vi "testAESDecryption-ECB-256.vi"(8 "error in (no error)":errorcluster, 11 "TestCase in":refnum<class "TestAES.lvclass">) -> (0 "error out":errorcluster, 3 "TestCase out":refnum<class "TestAES.lvclass">)   [LabVIEW 2021, in "TestAES.lvclass"]
uses:
  TestAES.lvclass
  C:/Program Files (x86)/National Instruments/LabVIEW 2021/vi.lib/addons/_JKI Toolkits/VI Tester/TestCase.llb/TestCase.lvclass
  TestAES.lvclass/TestAES.ctl
  <vilib>/addons/_JKI Toolkits/VI Tester/TestCase.llb/TestCase.lvclass
  <vilib>/Wiresmith Technology/VITAC (VI Tester Advanced Comparisons)/VITAC.lvlib
  Symmetric Encryption/dotNET Crypto Symmetric Encryption.lvlib
panel:
  out "Ciphertext in (hex)":string="Hello, World!"
  out "Key (hex)":string="01234567890"
  out "Expected plaintext (hex)":string
  out "Actual plaintext (hex)":string
  out "Expected plaintext":string
  out "Ciphertext in":string="Hello, World!"
  out "Actual plaintext":string
  out "Key":string="01234567890"
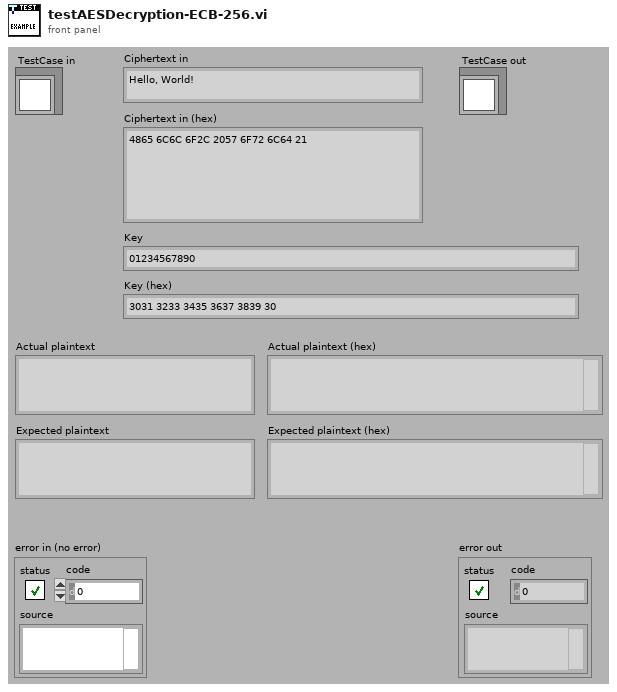
[diagram p1: front panel]
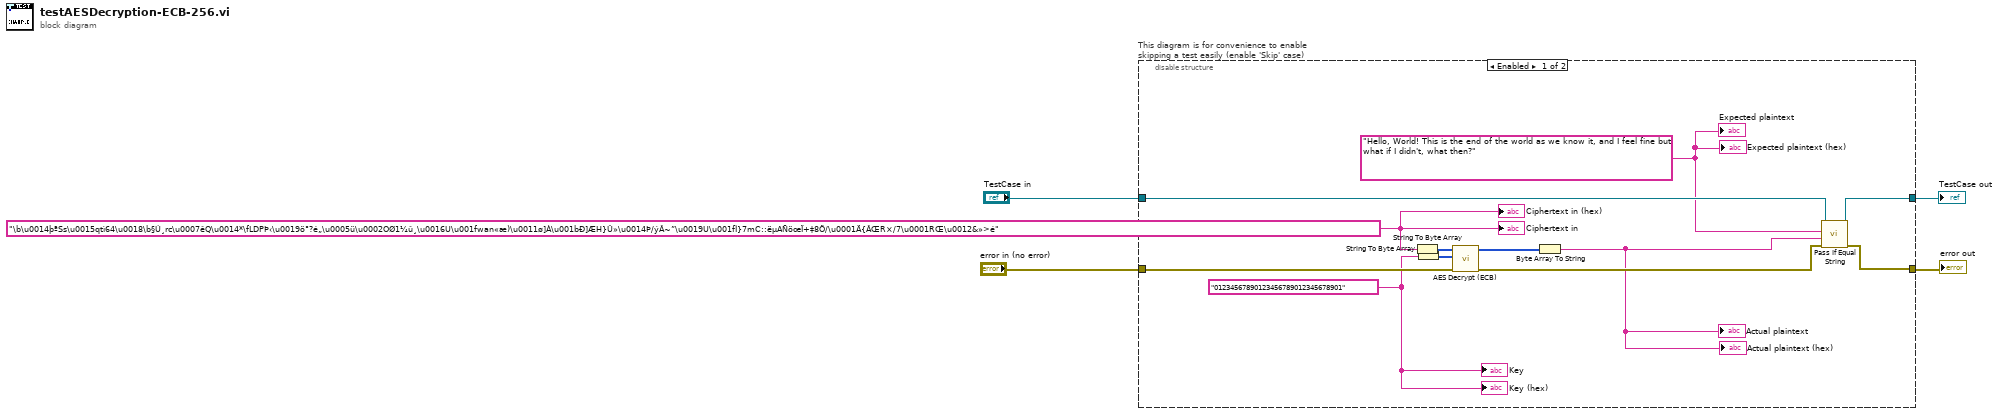
[diagram p0: block diagram]
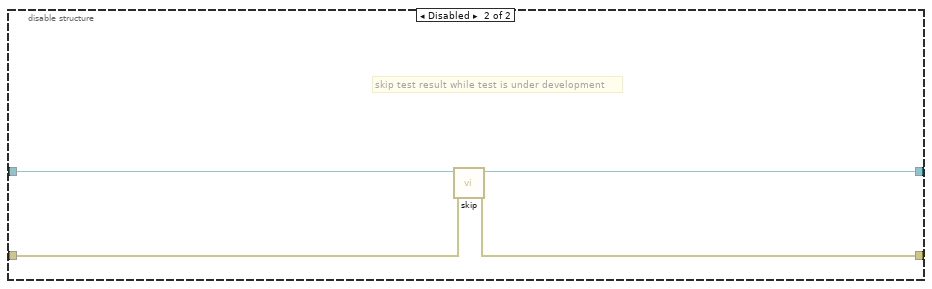
[diagram p2: hidden frame]
diagram:
  n1 = disable-structure "This diagram is for convenience to enable skipping a test easily (enable 'Skip' case)" shown="Enabled" {
    disable-tunnel: "TestCase in" -> [w16 w20]
    disable-tunnel: [w15 w18] -> w1
    disable-tunnel: [w14 w19] -> w3
    disable-tunnel: "error in (no error)" -> [w13 w17]
    frame Enabled {
      w10 = "Hello, World! This is the end of the world as we know it, and I feel fine but what if I didn't, what then?" ("Plaintext in")
      w9 = "01234567890123456789012345678901" ("Key")
      w8 = "\b\u0014þªSs\u0015qtì64\u0018\b§Ú¸rc\u0007êQ\u0014*\fLDPÞ‹\u0019ö°?é„\u0005ü\u0002OØ1¼û¸\u0016U\u001fwan«æ)\u0011ø]À\u001bÐ]ÆH}Û»\u0014Þ/ýÂ~”\u0019U\u001fÌ}7mC::ëµAÑöœÏ+‡8Ö/\u0001Ä{ÂŒR×/7\u0001RŒ\u0012&»>é" ("Plaintext in")
      n2 = String To Byte Array(string=w8) -> (unsigned byte array=w6:u8[])
      n3 = String To Byte Array(string=w9) -> (unsigned byte array=w5:u8[])
      n4 = call "AES Decrypt (ECB).vi"("error in (no error)"=w13, "Key"=w5, "Encrypted data in"=w6) -> ("error out"=w12:errorcluster, "Raw data out"=w11:u8[])  [unwired: 7 in]
      n5 = Byte Array To String(unsigned byte array=w11) -> (string=w7:string)
      "Actual plaintext" <- w7
      "Actual plaintext (hex)" <- w7
      n6 = call <vilib>:"Pass If Equal String.vi"("error in (no error)"=w12, "actual"=w7, "expected"=w10, "TestCase in"=w16) -> ("error out"=w14:errorcluster, "TestCase out"=w15:refnum<class "TestAES.lvclass">)  [unwired: 6 in]
      "Key" <- w9
      "Ciphertext in" <- w8
      "Expected plaintext" <- w10
      "Expected plaintext (hex)" <- w10
      "Key (hex)" <- w9
      "Ciphertext in (hex)" <- w8
    }
    frame Disabled {
      # "skip test result while test is under development"
      n7 = call <vilib>:"skip.vi"("error in (no error)"=w17, "TestCase in"=w20) -> ("error out"=w19:errorcluster, "TestCase out"=w18:refnum<class "TestAES.lvclass">)  [unwired: 8 in]
    }
  }
  "error out" <- w3
  "TestCase out" <- w1
